vi "CenterFinder - Copy.vi"() -> ()   [LabVIEW 2016]
uses:
  Control/ProcessCtl.ctl
  <vilib>/userdefined/High Color/IMAQdx.ctl
  <vilib>/vision/driver/NI_Vision_Acquisition_Software.lvlib
  <vilib>/vision/NI_Vision_Development_Module.lvlib
panel:
  out "Line Segment":T1
  in  "Edge Options":T2={"Edge Polarity"=2, "Kernel Size"=37, "Width"=5, "Minimum Edge Strength"=10.0, "Interpolation Type"=0, "Data Processing Method"=1} {"Edge Polarity" items=["All Edges", "Rising Edges", "Falling Edges"]; "Interpolation Type" items=["Zero Order"=0, "Bilinear"=1, "Bilinear Fixed"=4]; "Data Processing Method" items=["Average", "Median"]}
  out "LineEquation":cluster{"A":dbl, "B":dbl, "C":dbl}[](array[cluster])
  out "Array":T3(array[cluster])
  out "output cluster":cluster{"X":dbl, "Y":dbl, "Z":dbl}
  out "1":bool[](array[boolean])
  in  "Enum":enum16{"B2T", "L2R", "R2L", "T2B"}(ring)=enum."R2L"
  in  "Delete":bool
  in  "Retake":bool
  in  "Next":bool
  in  "Process":bool
  in  "Acquire":bool
  in  "stop":bool
  out "Image":T4(plugin-control)
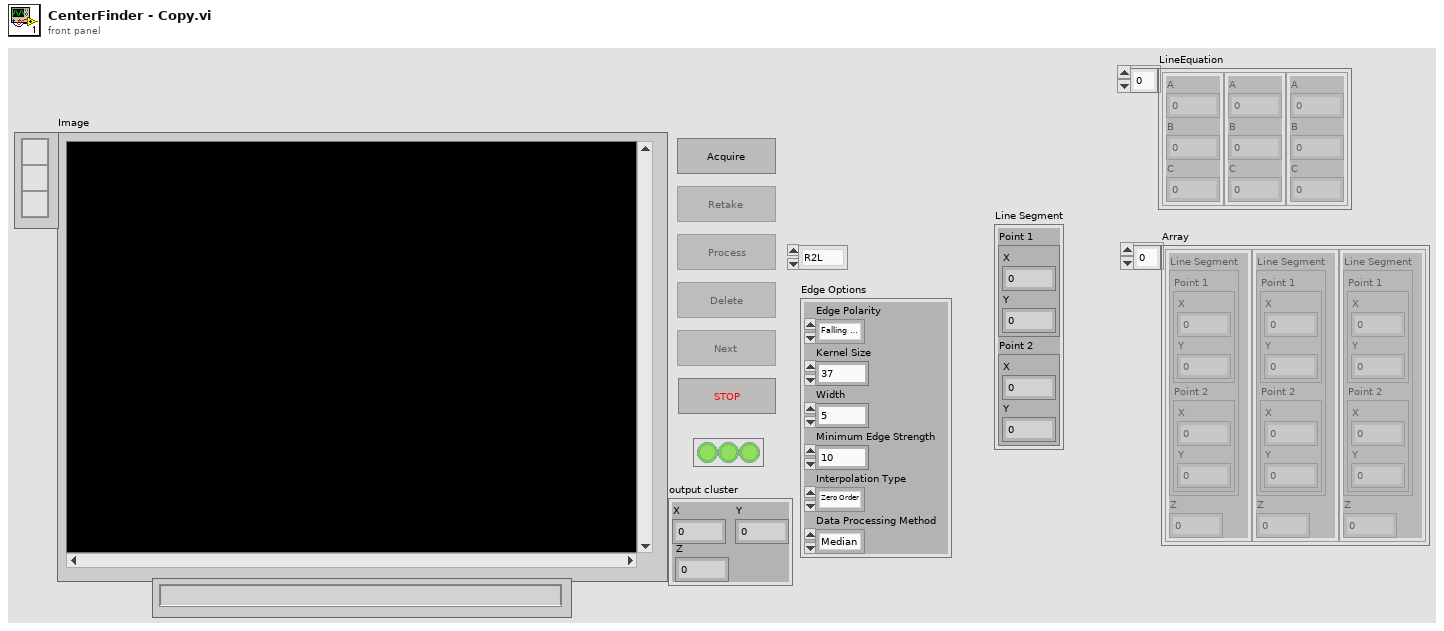
[diagram p1: front panel]
types:
  T1 = cluster{"Point 1":cluster{"X":sgl, "Y":sgl}, "Point 2":cluster{"X":sgl, "Y":sgl}}
  T2 = cluster{"Edge Polarity":u16, "Kernel Size":u32, "Width":u32, "Minimum Edge Strength":dbl, "Interpolation Type":u16, "Data Processing Method":u16}
  T3 = cluster{"Line Segment":cluster{"Point 1":cluster{"X":sgl, "Y":sgl}, "Point 2":cluster{"X":sgl, "Y":sgl}}, "Z":dbl}[]
  T4 = typedef "IMAQ Image.ctl" = refnum<image>
  T5 = typedef "IMAQdx.ctl" = refnum<k21>
  T6 = typedef "ProcessCtl.ctl" = enum16{"Idle", "Acquire", "Process", "Abort", "Initialize", "Wait"}
  T7 = enum8{"Enabled", "Disabled", "Disabled and Grayed Out"}
  T8 = cluster{"Line Segment":cluster{"Point 1":cluster{"X":sgl, "Y":sgl}, "Point 2":cluster{"X":sgl, "Y":sgl}}, "Z":dbl}
  T9 = typedef "Image Type" = u32
  T10 = typedef "IMAQ Line" = cluster{"Start X":i32, "Start Y":i32, "End X":i32, "End Y":i32}
  T11 = typedef "ROI Descriptor" = cluster{"Global Rectangle":i32[], "Contours":cluster{"ID":enum32{"External", "Internal"}, "Type":u32, "Coordinates":i32[]}[]}
  T12 = typedef "Edge New.ctl" = cluster{"Location (Pixel)":cluster{"X":sgl, "Y":sgl}, "Location (Real-World)":cluster{"X":sgl, "Y":sgl}, "Distance (Pixel)":dbl, "Distance (Real-World)":dbl, "Strength":dbl, "Noise":dbl, "Rising?":bool}
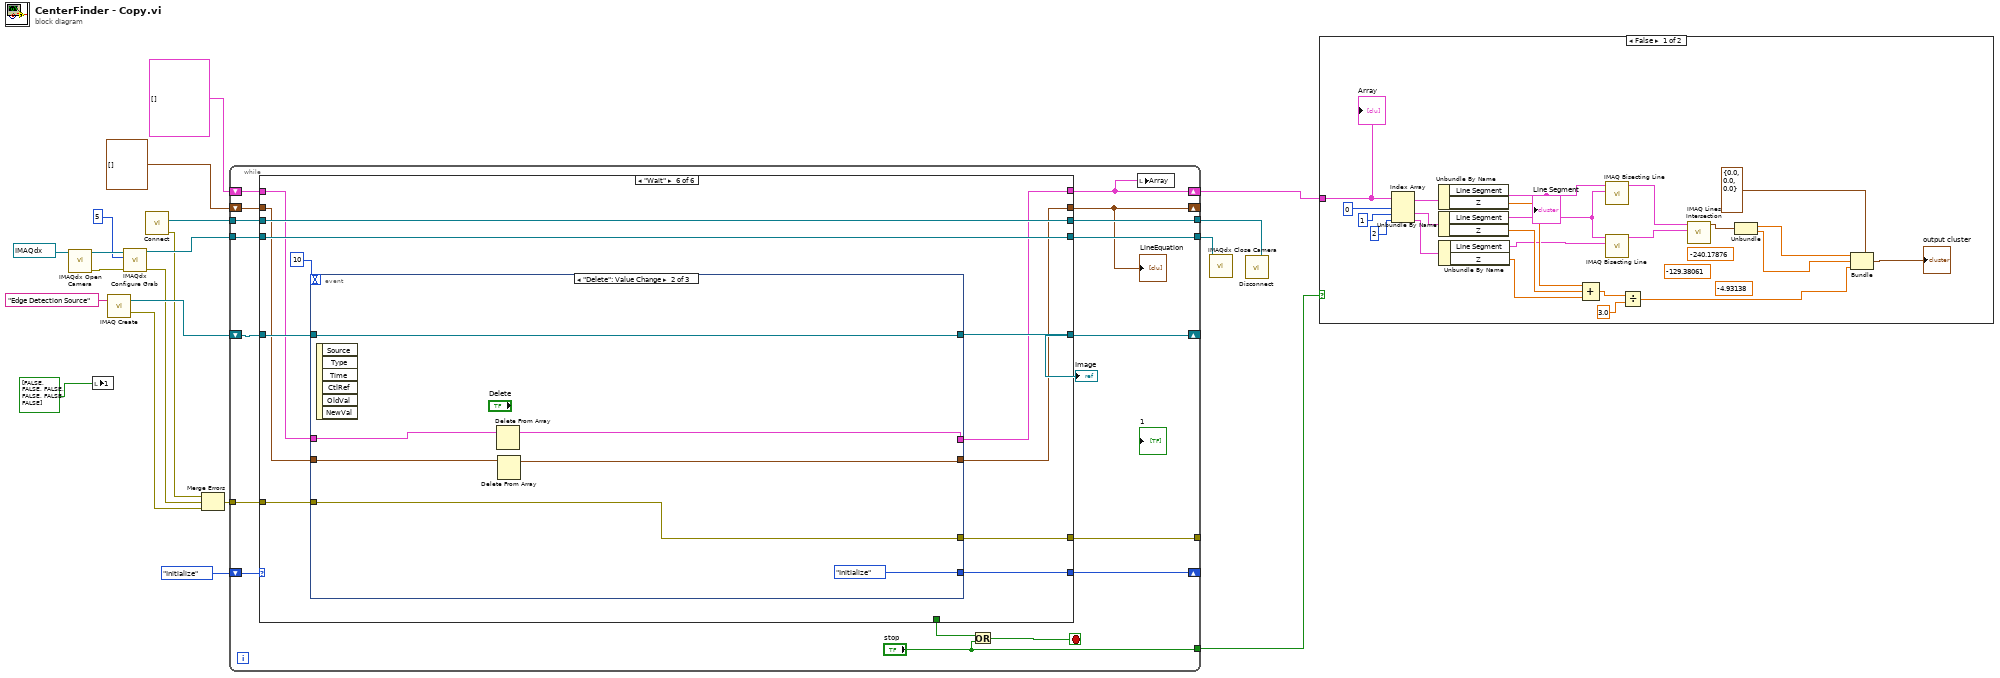
[diagram p0: block diagram]
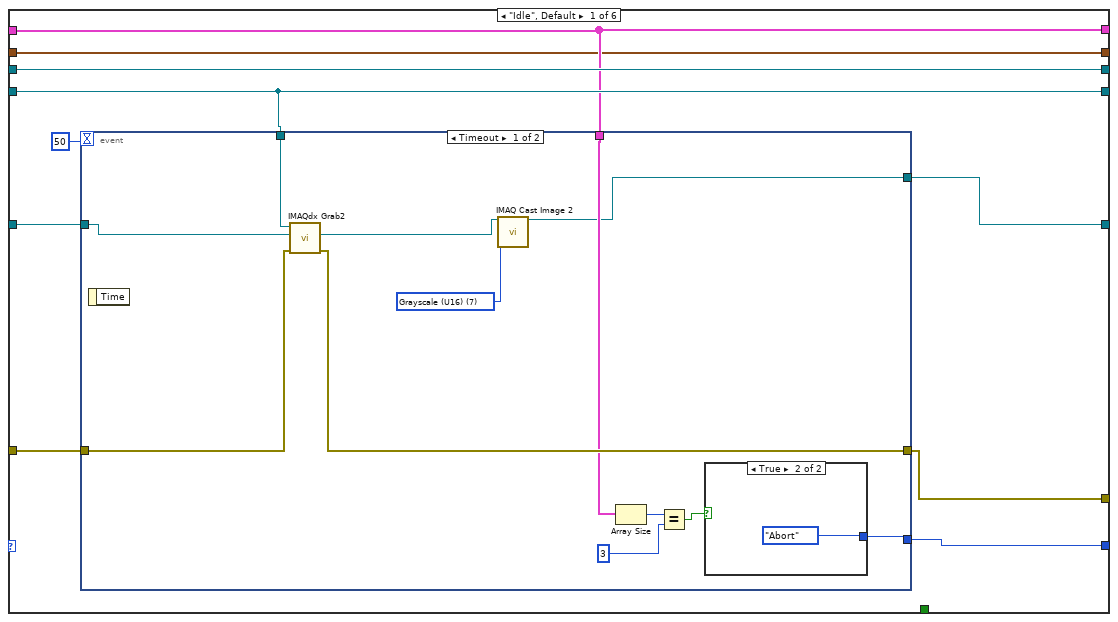
[diagram p3: hidden frame]
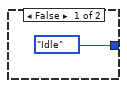
[diagram p4: hidden frame]
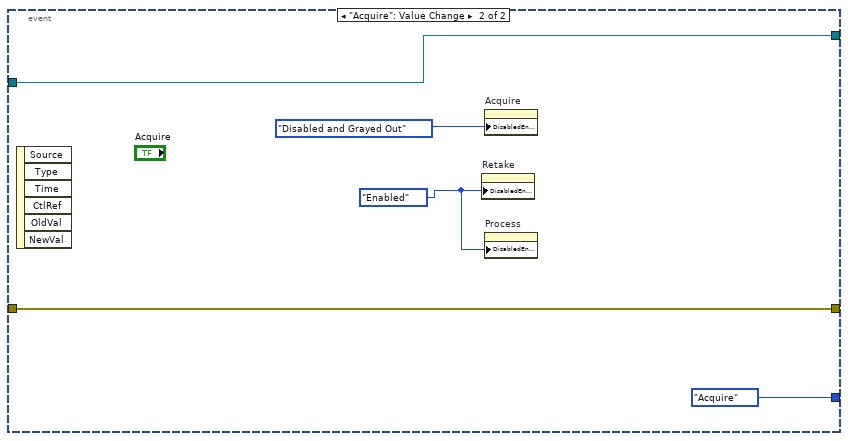
[diagram p5: hidden frame]
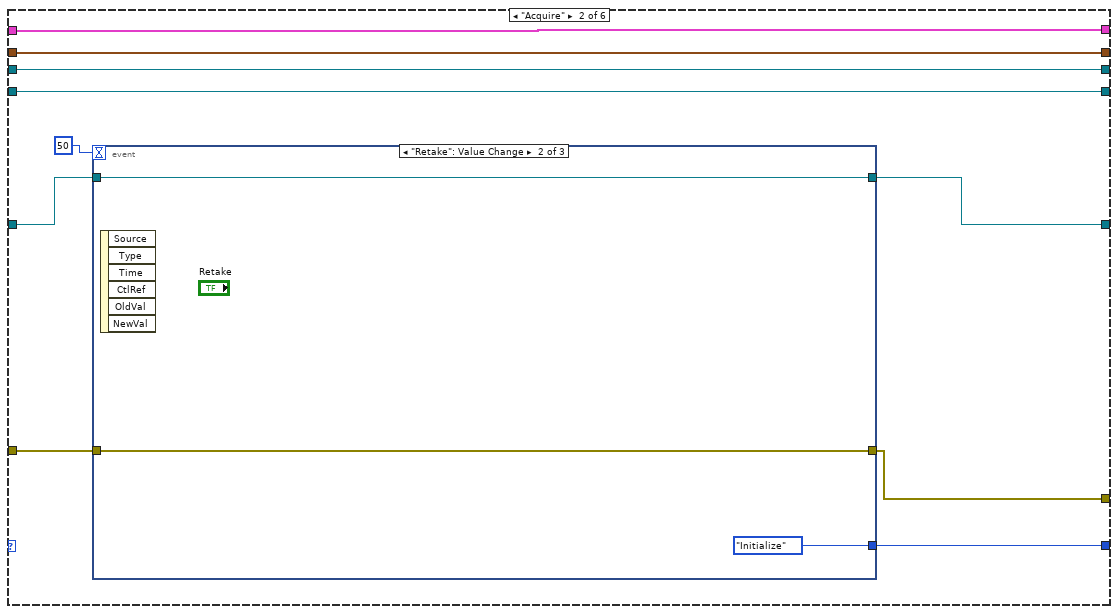
[diagram p6: hidden frame]
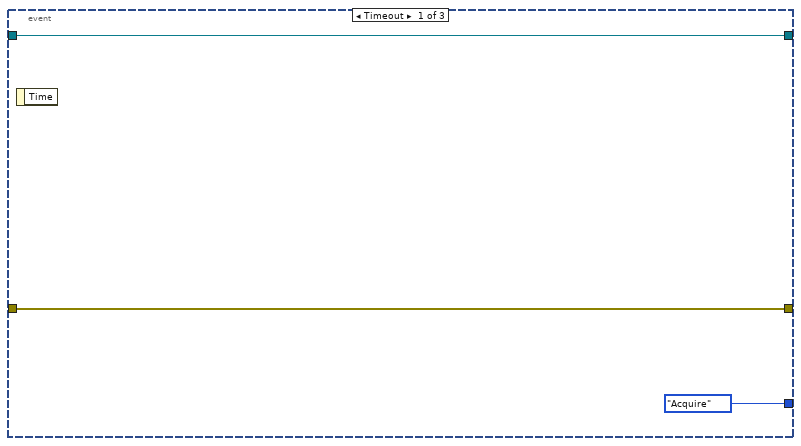
[diagram p7: hidden frame]
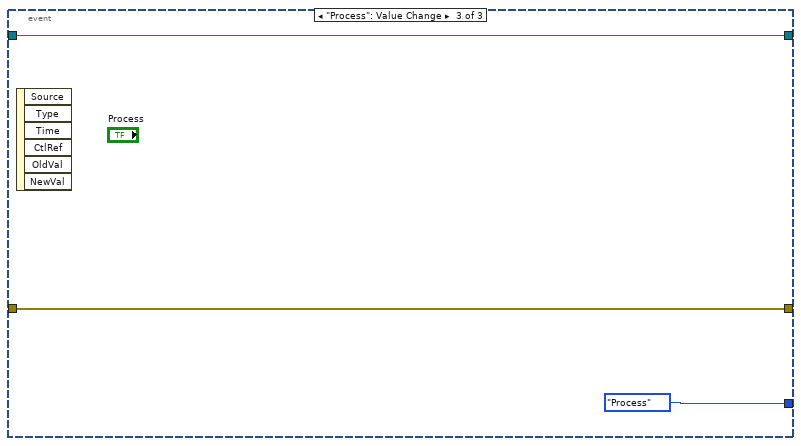
[diagram p8: hidden frame]
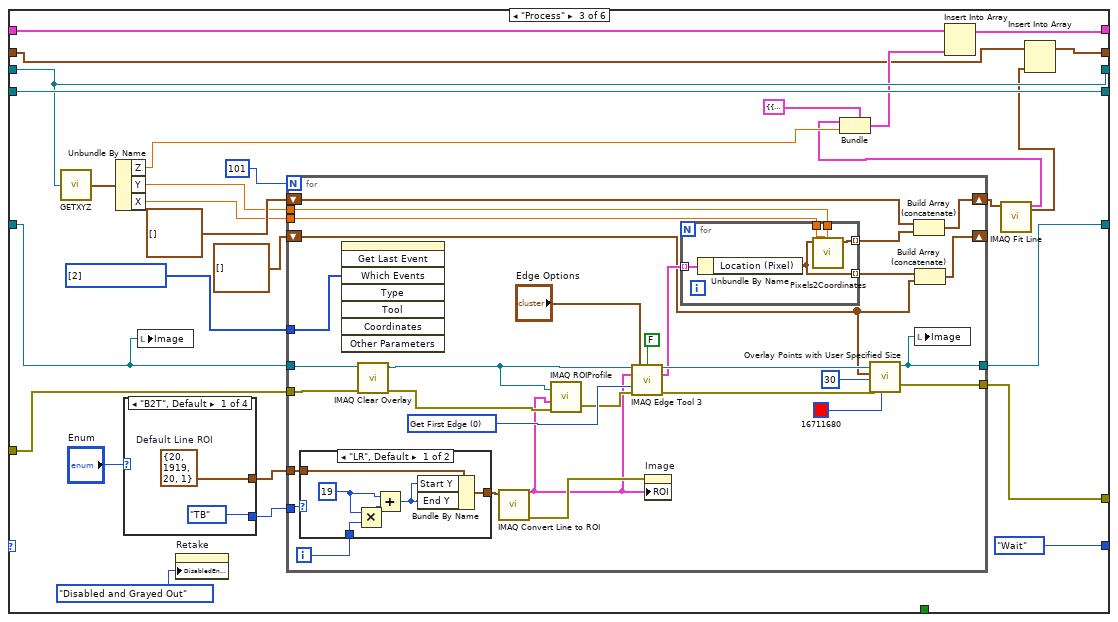
[diagram p9: hidden frame]
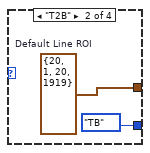
[diagram p10: hidden frame]
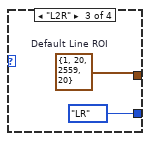
[diagram p11: hidden frame]
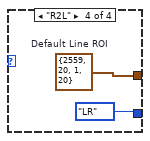
[diagram p12: hidden frame]
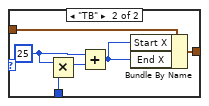
[diagram p13: hidden frame]
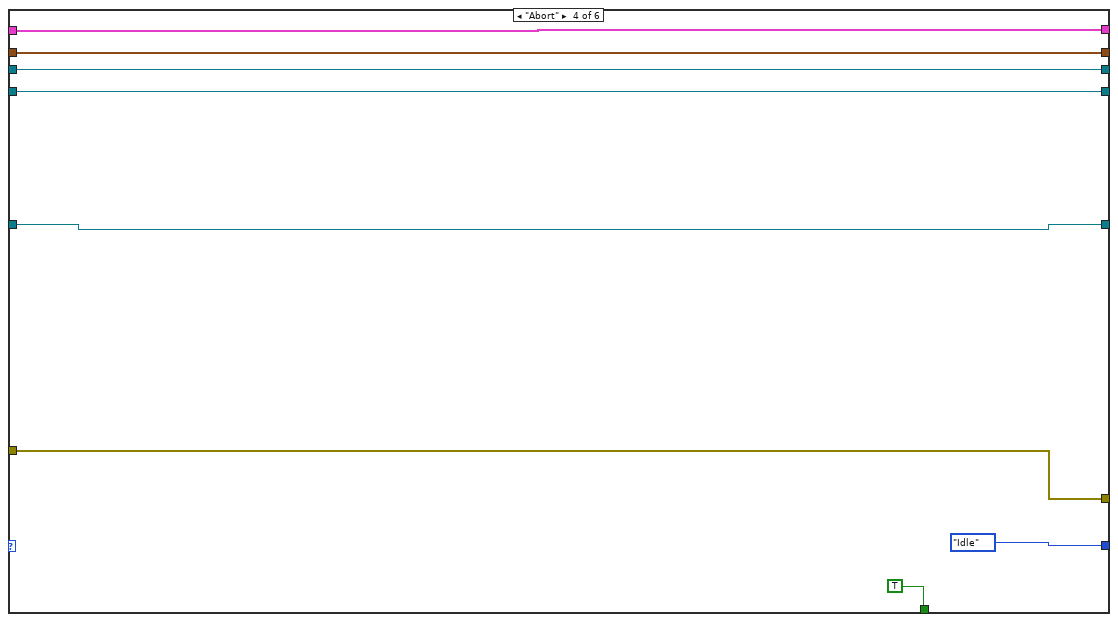
[diagram p14: hidden frame]
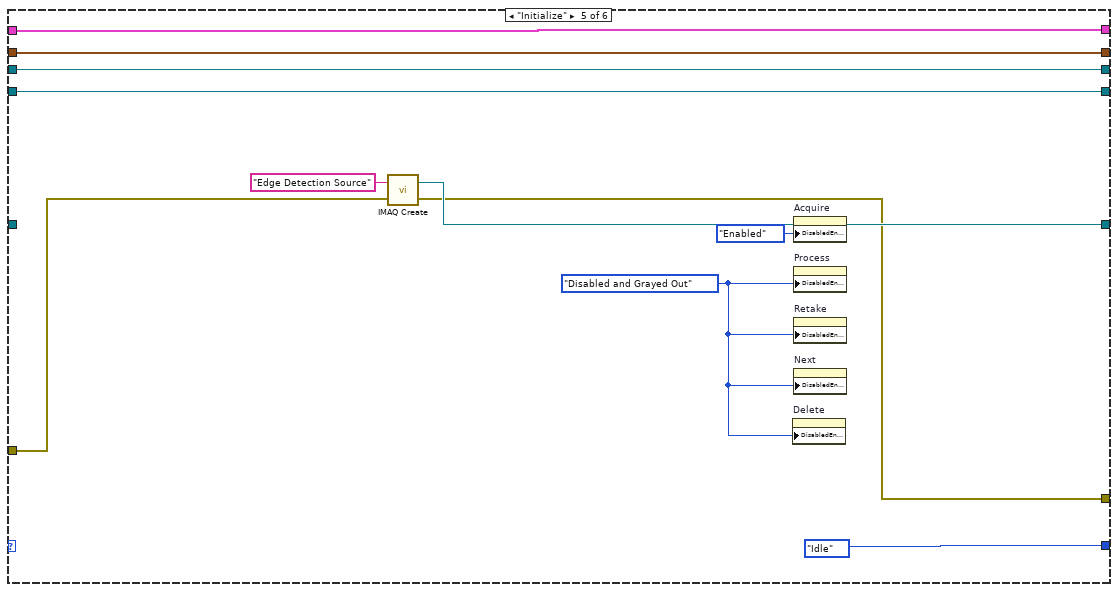
[diagram p15: hidden frame]
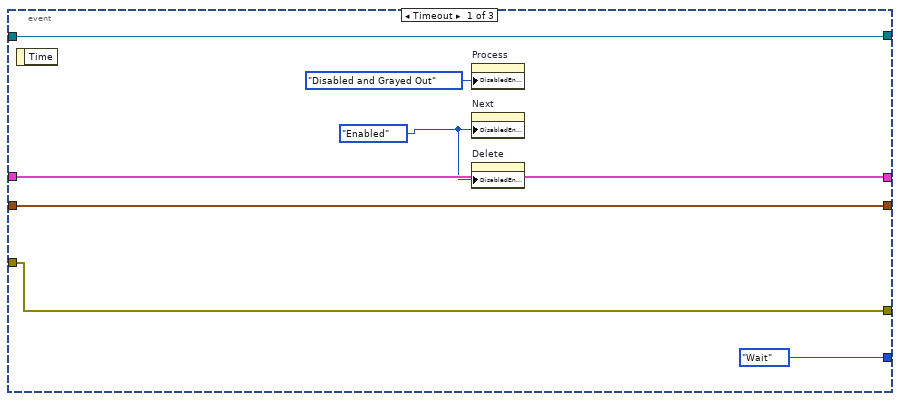
[diagram p16: hidden frame]
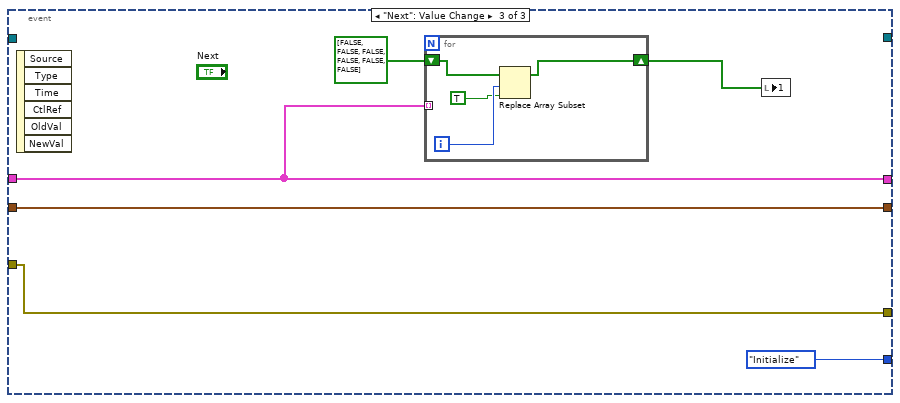
[diagram p17: hidden frame]
diagram:
  n1 = call <vilib>:"IMAQdx Open Camera.vi"("Session In"=T5 "cam0") -> ("error out"=w17:errorcluster, "Session Out"=w18:T5)  [unwired: 9 in]
  n2 = local write "1"(bool[] [FALSE, FALSE, FALSE, FALSE, FALSE, FALSE] ("1 2")) -> ()
  n3 = call "IMAQ Create"("Image Name"="Edge Detection Source") -> ("New Image"=w15:T4, "error out"=w8:errorcluster)  [unwired: 4 in]
  n4 = call <vilib>:"IMAQdx Configure Grab.vi"("error in"=w17, "Number of Buffers"=u32 5, "Session In"=w18) -> ("error out"=w9:errorcluster, "Session Out"=w19:T5)  [unwired: 7 in]
  n5 = call "Connect.vi"() -> ("error out"=w10:errorcluster, "controller"=w12:refnum<k24>)  [unwired: 10 in]
  n6 = Merge Errors(w10, w9, w8) -> (w7:errorcluster)
  n7 = while {
    tunnel: w19 -> [w28]
    tunnel: [w27] -> w13
    shift-right: [w34] -> _
    shift-left: w15 -> [w32]
    tunnel: w12 -> [w30]
    tunnel: [w29] -> w11
    tunnel: w7 -> [w37]
    shift-right: [w35] -> _
    shift-left: ProcessCtl."Initialize" -> [w36]
    tunnel: [w33] -> _
    shift-right: [w24] -> w3
    shift-left: T3 [] -> [w31]
    tunnel: ["stop"] -> w2
    shift-right: [w21] -> _
    shift-left: cluster{"A":dbl, "B":dbl, "C":dbl}[] [] ("Array 3") -> [w22]
    stop <- w25 stop-if-true
    n8 = case shown="\"Wait\"" w36 {
      tunnel: w37 -> [w47 w72 w112 w170 w183 w191]
      tunnel: [w43 w73 ProcessCtl."Wait" ProcessCtl."Idle" ProcessCtl."Idle" w197] -> w35
      tunnel: w32 -> [w46 w76 w94 w173 _ w199]
      tunnel: [w45 w75 w104 w173 w184 w198] -> w34
      tunnel: [w42 w71 w98 w170 w182 w192] -> w33
      tunnel: w31 -> [w39 w70 w100 w176 w181 w194]
      tunnel: [w39 w70 w99 w176 w181 w193] -> w24
      tunnel: w30 -> [w41 w69 w101 w175 w180 w196]
      tunnel: [w41 w69 w101 w175 w180 w196] -> w29
      tunnel: w28 -> [w40 w68 w102 w174 w179 w195]
      tunnel: [w40 w68 w102 w174 w179 w195] -> w27
      tunnel: [_ _ _ TRUE _ _] -> w26
      tunnel: w22 -> [w38 w67 w88 w169 w177 w189]
      tunnel: [w38 w67 w87 w169 w177 w188] -> w21
      frame "Idle", Default {
        n9 = event shown="[0] Timeout" {
          selector: _ -> [_ _]
          dyn-events: _ -> [_ _]
          timeout: 50 -> [_ _]
          tunnel: w47 -> [w59 w62]
          tunnel: w46 -> [w58 w64]
          tunnel: w40 -> [w57 _]
          tunnel: [w49 w64] -> w45
          tunnel: [w55 ProcessCtl."Acquire"] -> w43
          tunnel: [w56 w62] -> w42
          tunnel: w39 -> [w54 _]
          event Timeout {
            w50 = T9 7 items=["Grayscale (U8)", "Grayscale (I16)", "Grayscale (SGL)", "Complex (CSG)", "RGB (U32)", "HSL (U32)", "RGB (U64)", "Grayscale (U16)"] ("Image Type")
            n10 = event-data() -> ()  [unwired: 1 in, 1 out]
            n11 = call <vilib>:"IMAQdx Grab2.vi"("error in"=w59, "Image In"=w58, "Session In"=w57) -> ("error out"=w56:errorcluster, "Image Out"=w48:T4)  [unwired: 5 in, 2 out]
            n12 = call "IMAQ Cast Image 2"("Image Src"=w48, "Image Type"=w50) -> ("Image Dst Out"=w49:T4)  [unwired: 12 in, 1 out]
            n13 = Array Size(array=w54) -> (size(s)=w53:i32)
            n14 = Equal?(x=w53, y=3) -> (x = y?=w51:bool)
            n15 = case shown="True" w51 {
              tunnel: [ProcessCtl."Idle" ProcessCtl."Abort"] -> w55
              frame False {
              }
              frame True {
              }
            }
          }
          event "Acquire": Value Change {
            w63 = T7."Enabled" ("Disabled")
            n16 = event-data() -> ()  [unwired: 1 in, 6 out]
            n17 = property on="Retake" class="Bool"("DisabledEnum"=w63) -> ()  [unwired: 2 in, 2 out]
            n18 = property on="Acquire" class="Bool"("DisabledEnum"=T7."Disabled and Grayed Out" ("Disabled")) -> ()  [unwired: 2 in, 2 out]
            n19 = property on="Process" class="Bool"("DisabledEnum"=w63) -> ()  [unwired: 2 in, 2 out]
          }
        }
      }
      frame "Acquire" {
        n20 = event shown="[1] \"Retake\": Value Change" {
          selector: _ -> [_ _ _]
          dyn-events: _ -> [_ _ _]
          timeout: 50 -> [_ _ _]
          tunnel: w76 -> [w79 w80 w83]
          tunnel: [w79 w80 w83] -> w75
          tunnel: [ProcessCtl."Acquire" ProcessCtl."Initialize" ProcessCtl."Process"] -> w73
          tunnel: w72 -> [w77 w81 w84]
          tunnel: [w77 w81 w84] -> w71
          event Timeout {
            n21 = event-data() -> ()  [unwired: 1 in, 1 out]
          }
          event "Retake": Value Change {
            n22 = event-data() -> ()  [unwired: 1 in, 6 out]
          }
          event "Process": Value Change {
            n23 = event-data() -> ()  [unwired: 1 in, 6 out]
          }
        }
      }
      frame "Process" {
        w113 = i32[] [2] items=["No  event", "Click event", "Draw event", "Move event", "Size event", "Scroll event", "Activate event", "Close event", "Double click event"] ("Events list (all)")
        n24 = call "GETXYZ.vi"(".NET Refnum in"=w101) -> ("XYZ"=w107:cluster{"X":dbl, "Y":dbl, "Z":dbl})
        n25 = Unbundle By Name(w107) -> ("Z"=w91:dbl, "Y"=w106:dbl, "X"=w105:dbl)
        n26 = case shown="\"B2T\", Default" "Enum" {
          tunnel: [w115 w117 w118 w120] -> w110
          tunnel: [enum16{"LR", "TB"}."TB" enum16{"LR", "TB"}."TB" enum16{"LR", "TB"}."LR" enum16{"LR", "TB"}."LR"] -> w95
          frame "B2T", Default {
            w115 = T10 {"Start X"=20, "Start Y"=1919, "End X"=20, "End Y"=1}  # Default Line ROI
          }
          frame "T2B" {
            w117 = T10 {"Start X"=20, "Start Y"=1, "End X"=20, "End Y"=1919}  # Default Line ROI
          }
          frame "L2R" {
            w118 = T10 {"Start X"=1, "Start Y"=20, "End X"=2559, "End Y"=20}  # Default Line ROI
          }
          frame "R2L" {
            w120 = T10 {"Start X"=2559, "Start Y"=20, "End X"=1, "End Y"=20}  # Default Line ROI
          }
        }
        n27 = local write "Image"(w94) -> ()
        n28 = property on="Retake" class="Bool"("DisabledEnum"=T7."Disabled and Grayed Out" ("Disabled")) -> ()  [unwired: 2 in, 2 out]
        n29 = for {
          N: 101 -> [_]
          tunnel: w94 -> [w130]
          tunnel: w112 -> [w149]
          shift-right: [w140] -> w108
          shift-left: cluster{"X":sgl, "Y":sgl}[] [] -> [w142]
          tunnel: w113 -> [w134]
          tunnel: [w125] -> w104
          tunnel: [w139] -> w98
          tunnel: w110 -> [w137]
          tunnel: w106 -> [w136]
          tunnel: w105 -> [w135]
          tunnel: w95 -> [w132]
          shift-right: [w124] -> _
          shift-left: cluster{"X":sgl, "Y":sgl}[] [] -> [w122]
          i -> [w151]
          w148 = u16 0 items=["Get First Edge", "Get First + Last Edge", "Get All Edges", "Get Best Edge"] ("Process")
          n30 = case shown="\"LR\", Default" w132 {
            tunnel: w151 -> [w155 w163]
            tunnel: [w157 w159] -> w150
            tunnel: w137 -> [w156 w158]
            frame "LR", Default {
              w152 = 19
              n31 = Multiply(x=w152, y=w155) -> (x*y=w153:i32)
              n32 = Add(x=w152, y=w153) -> (x+y=w154:i32)
              n33 = Bundle By Name(cluster=w156, "Start Y"=w154, "End Y"=w154) -> (w157:T10)
            }
            frame "TB" {
              w161 = 25
              n34 = Multiply(x=w161, y=w163) -> (x*y=w162:i32)
              n35 = Add(x=w161, y=w162) -> (x+y=w160:i32)
              n36 = Bundle By Name(cluster=w158, "Start X"=w160, "End X"=w160) -> (w159:T10)
            }
          }
          n37 = invoke on="Image" class="ImageControl" method="Get Last Event"("Which Events"=w134) -> ()  [unwired: 7 in, 8 out]
          n38 = call "IMAQ Clear Overlay"("error in (no error)"=w149, "Image"=w130) -> ("error out"=w128:errorcluster, "Image Out"=w126:T4)  [unwired: 8 in]
          n39 = call "IMAQ Convert Line to ROI"("Line"=w150) -> ("error out"=w133:errorcluster, "ROI Descriptor"=w127:T11)  [unwired: 8 in]
          n40 = call "IMAQ ROIProfile"("error in (no error)"=w128, "ROI Descriptor"=w127, "Image"=w126) -> ("error out"=w129:errorcluster)  [unwired: 1 in, 4 out]
          n41 = call "IMAQ Edge Tool 3"("Image"=w126, "Edge Options"="Edge Options", "Optimized Mode"=FALSE, "ROI Descriptor"=w127, "Process"=w148, "error in (no error)"=w129) -> ("Image (duplicate)"=w145:T4, "Edge Information"=w131:T12[], "error out"=w144:errorcluster)  [unwired: 5 in, 2 out]
          n42 = property on="Image" class="ImageControl"(error in=w133, "ROI"=w127) -> ()  [unwired: 1 in, 2 out]
          n43 = for {
            tunnel: w131 -> [w168] mode=indexing
            tunnel: [w167] -> w141 mode=indexing
            tunnel: w136 -> [w166]
            tunnel: w135 -> [w165]
            tunnel: [w164] -> w123 mode=indexing
            n44 = Unbundle By Name(w168) -> ("Location (Pixel)"=w164:cluster{"X":sgl, "Y":sgl})
            n45 = call "Pixels2Coordinates.vi"("Y"=w166, "X"=w165, "Location (Pixel)"=w164) -> ("output cluster"=w167:cluster{"X":sgl, "Y":sgl})  [unwired: 8 in]
          }
          n46 = call "Overlay Points with User Specified Size.vi"("Color"=u32 16711680, "error in"=w144, "Point Diameter (5)"=30, "Points"=w122, "Image In"=w145) -> ("error out"=w139:errorcluster, "Image Out"=w125:T4)  [unwired: 5 in]
          n47 = Build Array (concatenate)(w142, w141) -> (w140:cluster{"X":sgl, "Y":sgl}[])
          n48 = Build Array (concatenate)(w123, w122) -> (w124:cluster{"X":sgl, "Y":sgl}[])
          n49 = local write "Image"(w125) -> ()
        }
        n50 = call "IMAQ Fit Line"("Points"=w108) -> ("Line Segment"=w90:T1, "Line Equation"=w86:cluster{"A":dbl, "B":dbl, "C":dbl})  [unwired: 5 in, 4 out]
        n51 = Bundle(cluster=T8 {"Line Segment"={"Point 1"={"X"=0.0, "Y"=0.0}, "Point 2"={"X"=0.0, "Y"=0.0}}, "Z"=0.0}, "Line Segment"=w90, "Z"=w91) -> (w89:T8)
        n52 = Insert Into Array(array=w100, new element=w89) -> (w99:T3)  [unwired: 1 in]
        n53 = Insert Into Array(array=w88, new element=w86) -> (w87:cluster{"A":dbl, "B":dbl, "C":dbl}[])  [unwired: 1 in]
      }
      frame "Abort" {
      }
      frame "Initialize" {
        w178 = T7."Disabled and Grayed Out" ("Disabled")
        n54 = call "IMAQ Create"("Image Name"="Edge Detection Source", "error in (no error)"=w183) -> ("New Image"=w184:T4, "error out"=w182:errorcluster)  [unwired: 3 in]
        n55 = property on="Delete" class="Bool"("DisabledEnum"=w178) -> ()  [unwired: 2 in, 2 out]
        n56 = property on="Acquire" class="Bool"("DisabledEnum"=T7."Enabled" ("Disabled")) -> ()  [unwired: 2 in, 2 out]
        n57 = property on="Process" class="Bool"("DisabledEnum"=w178) -> ()  [unwired: 2 in, 2 out]
        n58 = property on="Retake" class="Bool"("DisabledEnum"=w178) -> ()  [unwired: 2 in, 2 out]
        n59 = property on="Next" class="Bool"("DisabledEnum"=w178) -> ()  [unwired: 2 in, 2 out]
      }
      frame "Wait" {
        n60 = event shown="[1] \"Delete\": Value Change" {
          selector: _ -> [_ _ _]
          dyn-events: _ -> [_ _ _]
          timeout: 10 -> [_ _ _]
          tunnel: w199 -> [w206 w211 _]
          tunnel: [w206 w211 _] -> w198
          tunnel: [ProcessCtl."Wait" ProcessCtl."Initialize" ProcessCtl."Initialize"] -> w197
          tunnel: w194 -> [w204 w213 w217]
          tunnel: [w204 w212 w217] -> w193
          tunnel: [w203 w209 w218] -> w192
          tunnel: w191 -> [w203 w209 w218]
          tunnel: w189 -> [w200 w208 w214]
          tunnel: [w200 w207 w214] -> w188
          event Timeout {
            w201 = T7."Enabled" ("Disabled")
            n61 = event-data() -> ()  [unwired: 1 in, 1 out]
            n62 = property on="Process" class="Bool"("DisabledEnum"=T7."Disabled and Grayed Out" ("Disabled")) -> ()  [unwired: 2 in, 2 out]
            n63 = property on="Next" class="Bool"("DisabledEnum"=w201) -> ()  [unwired: 2 in, 2 out]
            n64 = property on="Delete" class="Bool"("DisabledEnum"=w201) -> ()  [unwired: 2 in, 2 out]
          }
          event "Delete": Value Change {
            n65 = event-data() -> ()  [unwired: 1 in, 6 out]
            n66 = Delete From Array(array=w213) -> (array with subset deleted=w212:T3)  [unwired: 2 in, 1 out]
            n67 = Delete From Array(array=w208) -> (array with subset deleted=w207:cluster{"A":dbl, "B":dbl, "C":dbl}[])  [unwired: 2 in, 1 out]
          }
          event "Next": Value Change {
            n68 = event-data() -> ()  [unwired: 1 in, 6 out]
            n69 = for {
              tunnel: w217 -> [_] mode=indexing
              shift-right: [w220] -> w215
              shift-left: bool[] [FALSE, FALSE, FALSE, FALSE, FALSE, FALSE] ("1 2") -> [w223]
              i -> [w222]
              n70 = Replace Array Subset(array=w223, new element=TRUE, index=w222) -> (w220:bool[])
            }
            n71 = local write "1"(w215) -> ()
          }
        }
      }
    }
    "Image" <- w34
    "LineEquation" <- w21
    n72 = Or(x=w26, y="stop") -> (x .or. y?=w25:bool)
    n73 = local write "Array"(w24) -> ()
  }
  n74 = call <vilib>:"IMAQdx Close Camera.vi"("Session In"=w13) -> ()  [unwired: 10 in, 1 out]
  n75 = call "Disconnect.vi"("controller"=w11) -> ()  [unwired: 10 in, 1 out]
  n76 = case shown="False" w2 {
    tunnel: w3 -> [w246 _]
    frame False {
      (unwired) -4.93138
      (unwired) -129.38061
      (unwired) -240.17876
      n77 = Index Array(array=w246, index #1=0, index #2=1, index #3=2) -> (element #1=w242:T8, element #2=w241:T8, element #3=w240:T8)
      n78 = Unbundle By Name(w242) -> ("Line Segment"=w229:T1, "Z"=w237:dbl)
      "Line Segment" <- w229
      n79 = Unbundle By Name(w241) -> ("Line Segment"=w227:T1, "Z"=w236:dbl)
      n80 = Unbundle By Name(w240) -> ("Line Segment"=w228:T1, "Z"=w235:dbl)
      n81 = Compound Arithmetic op=ADD(w237, w236, w235) -> (w234:dbl)
      n82 = call "IMAQ Bisecting Line"("Line 2"=w228, "Line 1"=w227) -> ("Bisecting Line"=w238:T1)  [unwired: 8 in, 1 out]
      n83 = call "IMAQ Bisecting Line"("Line 2"=w227, "Line 1"=w229) -> ("Bisecting Line"=w239:T1)  [unwired: 8 in, 1 out]
      n84 = Divide(x=w234, y=3.0) -> (x/y=w225:dbl)
      n85 = call "IMAQ Lines Intersection"("Line 2"=w238, "Line 1"=w239) -> ("Intersection Point"=w232:cluster{"X":sgl, "Y":sgl})  [unwired: 7 in, 2 out]
      n86 = Unbundle(w232) -> ("X"=w224:sgl, "Y"=w226:sgl)
      n87 = Bundle(cluster=cluster{"X":dbl, "Y":dbl, "Z":dbl} {"X"=0.0, "Y"=0.0, "Z"=0.0}, "X"=w224, "Y"=w226, "Z"=w225) -> (→"output cluster":cluster{"X":dbl, "Y":dbl, "Z":dbl})
      "Array" <- w246
    }
    frame True {
    }
  }
